vi "BuildCTRL1Word.vi"(11 "Configure NAU7802 CTRL1":T1) -> (3 "string":string)   [LabVIEW 2020, in "CTI-Peripheral.lvlib" / "Adafruit NAU7802 24bit Strain Gauge.lvclass"]
uses:
  Adafruit NAU7802 24bit Strain Gauge.lvclass
  ConfigDataCTRL1.ctl
  NAU7802PGA.ctl
  NAU7802LDOVoltage.ctl
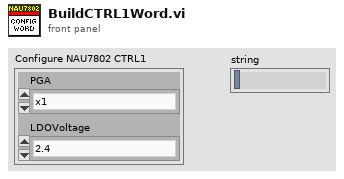
[diagram p1: front panel]
types:
  T1 = typedef "CTI-Peripheral.lvlib/Adafruit NAU7802 24bit Strain Gauge.lvclass/ConfigDataCTRL1.ctl" = cluster{"PGA":T2, "LDOVoltage":T3}
  T2 = typedef "CTI-Peripheral.lvlib/Adafruit NAU7802 24bit Strain Gauge.lvclass/NAU7802PGA.ctl" = enum16{"x1", "x2", "x4", "x8", "x16", "x32", "x64", "x128"}
  T3 = typedef "CTI-Peripheral.lvlib/Adafruit NAU7802 24bit Strain Gauge.lvclass/NAU7802LDOVoltage.ctl" = enum16{"2.4", "2.7", "3.0", "3.3", "3.6", "3.9", "4.2", "4.5"}
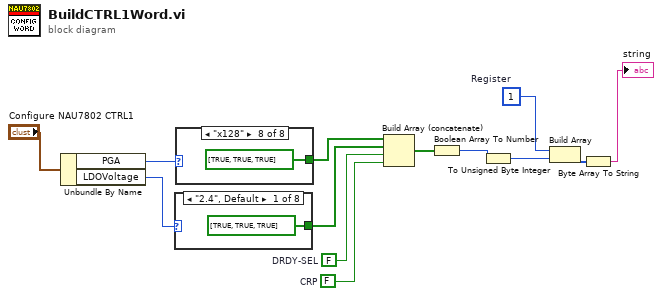
[diagram p0: block diagram]
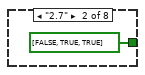
[diagram p2: hidden frame]
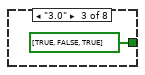
[diagram p3: hidden frame]
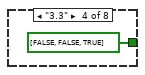
[diagram p4: hidden frame]
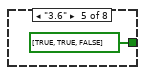
[diagram p5: hidden frame]
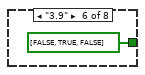
[diagram p6: hidden frame]
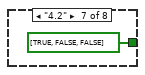
[diagram p7: hidden frame]
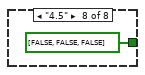
[diagram p8: hidden frame]
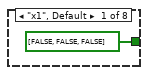
[diagram p9: hidden frame]
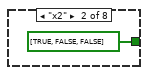
[diagram p10: hidden frame]
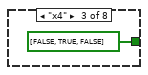
[diagram p11: hidden frame]
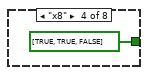
[diagram p12: hidden frame]
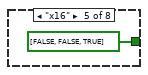
[diagram p13: hidden frame]
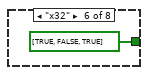
[diagram p14: hidden frame]
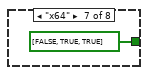
[diagram p15: hidden frame]
diagram:
  w2 = FALSE  # CRP
  w3 = FALSE  # DRDY-SEL
  w6 = u8 1  # Register
  n1 = Unbundle By Name("Configure NAU7802 CTRL1") -> ("PGA"=w8:T2, "LDOVoltage"=w9:T3)
  n2 = case shown="\"2.4\", Default" w9 {
    tunnel: [bool[] [TRUE, TRUE, TRUE] bool[] [FALSE, TRUE, TRUE] bool[] [TRUE, FALSE, TRUE] bool[] [FALSE, FALSE, TRUE] bool[] [TRUE, TRUE, FALSE] bool[] [FALSE, TRUE, FALSE] bool[] [TRUE, FALSE, FALSE] bool[] [FALSE, FALSE, FALSE]] -> w11
    frame "2.4", Default {
    }
    frame "2.7" {
    }
    frame "3.0" {
    }
    frame "3.3" {
    }
    frame "3.6" {
    }
    frame "3.9" {
    }
    frame "4.2" {
    }
    frame "4.5" {
    }
  }
  n3 = case shown="\"x128\"" w8 {
    tunnel: [bool[] [FALSE, FALSE, FALSE] bool[] [TRUE, FALSE, FALSE] bool[] [FALSE, TRUE, FALSE] bool[] [TRUE, TRUE, FALSE] bool[] [FALSE, FALSE, TRUE] bool[] [TRUE, FALSE, TRUE] bool[] [FALSE, TRUE, TRUE] bool[] [TRUE, TRUE, TRUE]] -> w10
    frame "x1", Default {
    }
    frame "x2" {
    }
    frame "x4" {
    }
    frame "x8" {
    }
    frame "x16" {
    }
    frame "x32" {
    }
    frame "x64" {
    }
    frame "x128" {
    }
  }
  n4 = Build Array (concatenate)(w10, w11, w3, w2) -> (w5:bool[])
  n5 = Boolean Array To Number(Boolean array=w5) -> (number=w4:u32)
  n6 = To Unsigned Byte Integer(number=w4) -> (unsigned 8bit integer=w1:u8)
  n7 = Build Array(w6, w1) -> (w12:u8[])
  n8 = Byte Array To String(unsigned byte array=w12) -> (string=→"string":string)
